vi "onDisconnection.vi"(8 "error in (no error)":errorcluster, 11 "Connection":refnum<class "Connection.lvclass">) -> (0 "error out":errorcluster, 3 "No connection":refnum<class "Connection.lvclass">)   [LabVIEW 2013, in "MQTT_Connection.lvlib" / "Connection.lvclass"]
uses:
  Connection.lvclass
  Connection.lvclass/Connection.ctl
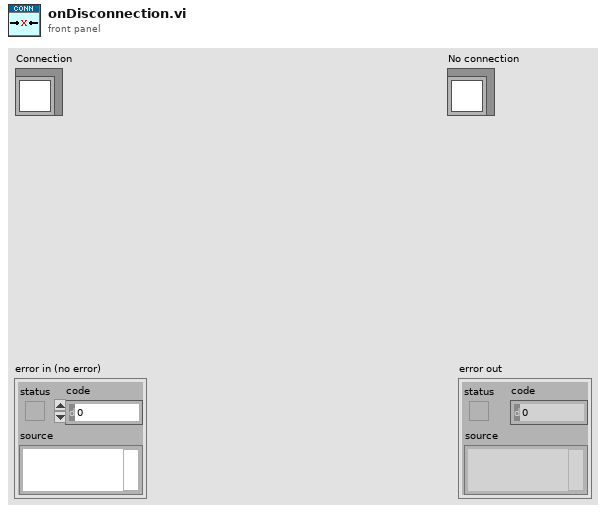
[diagram p1: front panel]
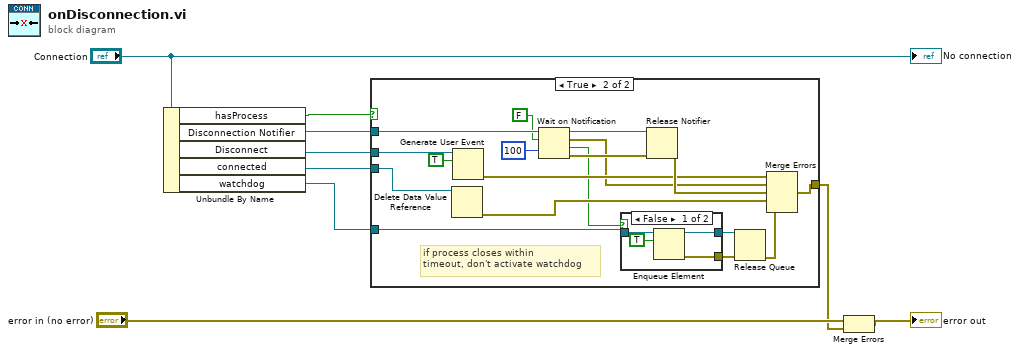
[diagram p0: block diagram]
diagram:
  n1 = Unbundle By Name("Connection") -> ("hasProcess"=w3:bool, "Disconnection Notifier"=w8:refnum<notifier>, "Disconnect"=w9:refnum<user-event>, "connected"=w2:refnum<data-value>, "watchdog"=w1:refnum<queue>)
  n2 = case shown="True" w3 {
    tunnel: w9 -> [_ w27]
    tunnel: w8 -> [_ w26]
    tunnel: [_ w19] -> w5
    tunnel: w2 -> [_ w18]
    tunnel: w1 -> [_ w14]
    frame False {
    }
    frame True {
      # "if process closes within\ntimeout, don't activate watchdog"
      n3 = Delete Data Value Reference(data value reference=w18) -> (error out=w17:errorcluster)  [unwired: 1 in, 1 out]
      n4 = Generate User Event(user event=w27, event data cluster=TRUE ("event data")) -> (error out=w20:errorcluster)  [unwired: 2 in, 1 out]
      n5 = Wait on Notification(notifier=w26, ignore previous (F)=FALSE, timeout in ms (-1)=100) -> (notifier out=w22:refnum<notifier>, notification=w15:errorcluster, timed out?=w10:bool, error out=w16:errorcluster)  [unwired: 1 in]
      n6 = case shown="False" w10 {
        tunnel: w14 -> [w31 w32]
        tunnel: [w30 w32] -> w13
        tunnel: [w28 _] -> w12
        frame False {
          n7 = Enqueue Element(queue=w31, element=TRUE) -> (queue out=w30:refnum<queue>, error out=w28:errorcluster)  [unwired: 2 in, 1 out]
        }
        frame True {
        }
      }
      n8 = Release Notifier(notifier=w22, error in (no error)=w16) -> (error out=w21:errorcluster)  [unwired: 1 in, 2 out]
      n9 = Release Queue(queue=w13, error in (no error)=w12) -> (error out=w11:errorcluster)  [unwired: 1 in, 2 out]
      n10 = Merge Errors(w20, w15, w21, w17, w11) -> (w19:errorcluster)
    }
  }
  n11 = Merge Errors("error in (no error)", w5) -> (→"error out":errorcluster)
  "No connection" <- "Connection"
